vi "ExpGlobals.vi"() -> ()   [LabVIEW 2017]
panel:
  in  "Cleanup interval in seconds":dbl
  in  "last experiment cleanup time":timestamp
  out "ExperimentInfoByID":variant
  out "Matlab Enviroment Started":bool
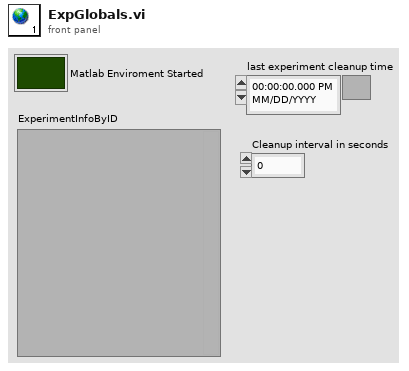
[diagram p1: front panel]
diagram:
